vi "FindClosestGObject.vi"(8 "error in (no error)":errorcluster, 10 "Coordinates":T1, 11 "List of GObjects":refnum<vi>[](array[refnum])) -> (0 "error out":errorcluster, 3 "Closest GObject":refnum<vi>)   [LabVIEW 2012]
doc: "Finds the closest GObject (input Array) from the coordinates."
uses:
  <vilib>/Utility/miscctls.llb/LVPoint32TypeDef.ctl
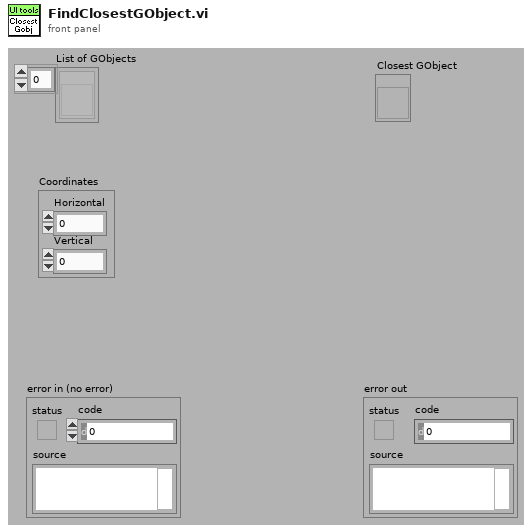
[diagram p1: front panel]
types:
  T1 = typedef "LVPoint32TypeDef.ctl" = cluster{"Horizontal":i32, "Vertical":i32}
  T2 = typedef "LVPositionTypeDef.ctl" = cluster{"Left":i32, "Top":i32}
  T3 = typedef "LVBoundsTypeDef.ctl" = cluster{"Width":u32, "Height":u32}
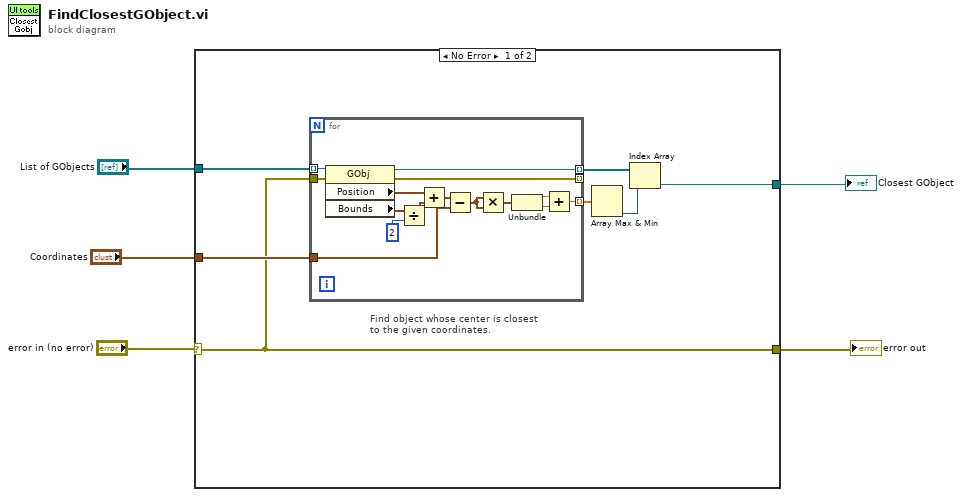
[diagram p0: block diagram]
diagram:
  n1 = case shown="No Error" "error in (no error)" {
    selector: "error in (no error)" -> [w6 w28]
    tunnel: "List of GObjects" -> [w9 _]
    tunnel: "Coordinates" -> [w8 _]
    tunnel: [w7 _] -> w4
    tunnel: [w6 w28] -> w2
    frame No Error {
      # "Find object whose center is closest\nto the given coordinates."
      n2 = for {
        tunnel: w9 -> [w27] mode=indexing
        tunnel: w8 -> [w21]
        tunnel: [w16] -> w12 mode=indexing
        tunnel: [w15] -> w11 mode=indexing
        tunnel: w6 -> [w14]
        tunnel: [w13] -> _ mode=indexing
        n3 = property class="GObj"(reference=w27, error in=w14) -> (reference out=w15:refnum<vi>, error out=w13:errorcluster, "Position"=w24:T2, "Bounds"=w26:T3)
        n4 = Divide(x=w26, y=2) -> (x/y=w23:cluster{"Width":dbl, "Height":dbl})
        n5 = Add(x=w24, y=w23) -> (x+y=w22:cluster{dbl, dbl})
        n6 = Subtract(x=w22, y=w21) -> (x-y=w20:cluster{dbl, dbl})
        n7 = Multiply(x=w20, y=w20) -> (x*y=w19:cluster{dbl, dbl})
        n8 = Unbundle(w19) -> (w17:dbl, w18:dbl)
        n9 = Add(x=w17, y=w18) -> (x+y=w16:dbl)
      }
      n10 = Array Max & Min(array=w12) -> (min index (indices)=w10:i32)  [unwired: 3 out]
      n11 = Index Array(array=w11, index=w10) -> (element=w7:refnum<vi>)
    }
    frame Error {
    }
  }
  "error out" <- w2
  "Closest GObject" <- w4
